vi "Init.vi"(9 "Dt":dbl, 10 "Size":i32, 11 "Fit Exponential in":refnum<class "Fit Exponential.lvclass">) -> (3 "Fit Exponential out":refnum<class "Fit Exponential.lvclass">)   [LabVIEW 2016, in "Exponential Fit Library.lvlib" / "Fit Exponential.lvclass"]
uses:
  Fit Exponential.lvclass
  Fit Exponential.lvclass/Fit Exponential.ctl
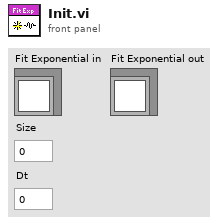
[diagram p1: front panel]
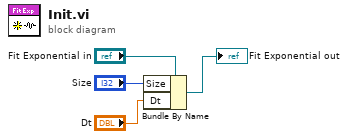
[diagram p0: block diagram]
diagram:
  n1 = Bundle By Name(cluster="Fit Exponential in", "Size"="Size", "Dt"="Dt") -> (→"Fit Exponential out":refnum<class "Fit Exponential.lvclass">)
